vi "close.vi"(8 "error in (no error)":errorcluster, 11 "TestScenarioFactory in":refnum<class "TestScenarioFactory.lvclass">) -> (0 "error out":errorcluster, 3 "TestScenarioFactory out":refnum<class "TestScenarioFactory.lvclass">)   [LabVIEW 2015, in "TestScenarioFactory.lvclass"]
uses:
  TestScenarioFactory.lvclass
  TestScenarioFactory.lvclass/TestScenarioFactory.ctl
  TestLog/ITestLog/ITestLog.lvclass
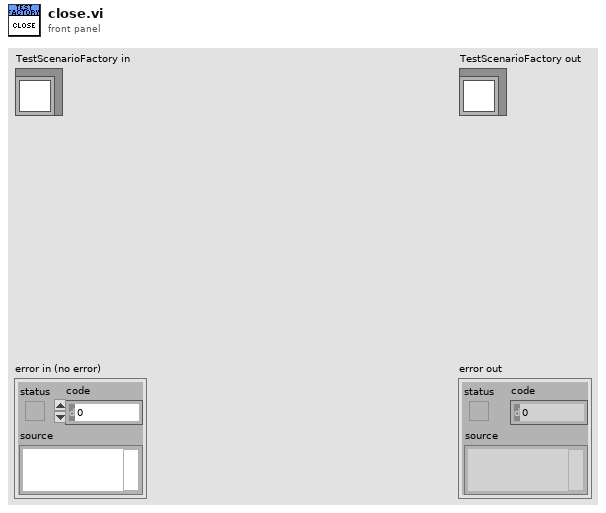
[diagram p1: front panel]
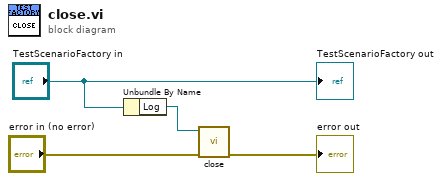
[diagram p0: block diagram]
diagram:
  n1 = Unbundle By Name("TestScenarioFactory in") -> ("Log"=w3:refnum<class "ITestLog.lvclass">)
  n2 = call-dynamic "close.vi"("error in (no error)"="error in (no error)", "ITestLog in"=w3) -> ("error out"=→"error out":errorcluster)  [unwired: 8 in, 1 out]
  "TestScenarioFactory out" <- "TestScenarioFactory in"
